vi "DAQ device.vi"(11 "data":dbl) -> ()   [LabVIEW 2025]
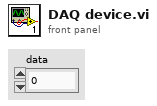
[diagram p1: front panel]
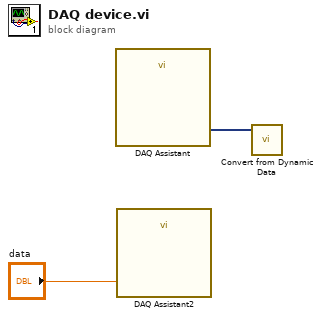
[diagram p0: block diagram]
diagram:
  n1 = call "DAQ Assistant"() -> ("data"=w1:dynamicdata)  [unwired: 17 in, 2 out]
  n2 = call "DAQ Assistant2"("data"="data") -> ()  [unwired: 17 in, 2 out]
  n3 = call "Convert from Dynamic Data"("Dynamic Data Type"=w1) -> ()  [unwired: 3 in, 1 out]
